vi "Get Background Settings.vi"(8 "error in":errorcluster, 9 "BigMAQ":refnum<class "BigMAQ.lvclass">, 11 "Inset in":refnum<class "Inset.lvclass">) -> (0 "error out":errorcluster, 1 "Background.Page":i32, 2 "Background.Range":cluster{sgl, sgl}, 3 "Inset out":refnum<class "Inset.lvclass">, 4 "status":bool)   [LabVIEW 2019, in "Inset.lvclass"]
uses:
  Inset.lvclass
  BigMAQ/BigMAQ.lvclass
  Inset.lvclass/Inset.ctl
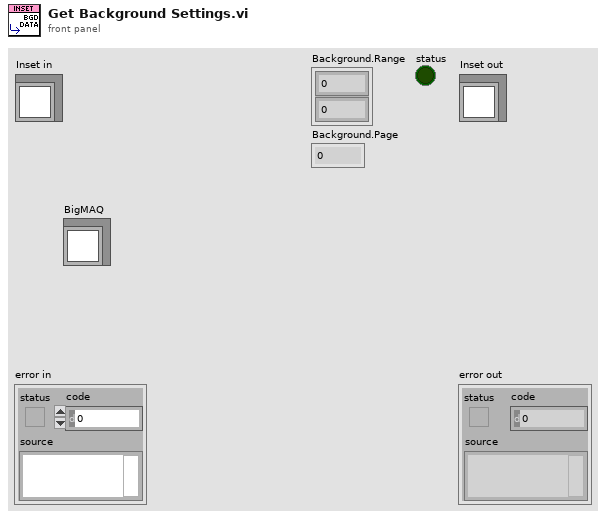
[diagram p1: front panel]
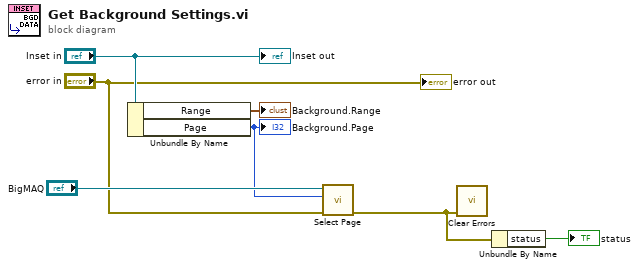
[diagram p0: block diagram]
diagram:
  n1 = Unbundle By Name("Inset in") -> ("Range"=→"Background.Range":cluster{sgl, sgl}, "Page"=w4:i32)
  "Background.Page" <- w4
  n2 = call "Select Page.vi"("error in (no error)"="error in", "Page"=w4, "BigMAQ in"="BigMAQ") -> ("error out"=w1:errorcluster)  [unwired: 6 in, 2 out]
  n3 = call <vilib>:"Clear Errors.vi"("error in (no error)"=w1) -> ()  [unwired: 5 in, 2 out]
  n4 = Unbundle By Name(w1) -> ("status"=→"status":bool)
  "error out" <- "error in"
  "Inset out" <- "Inset in"
